vi "MultiScanDrift.vi"() -> ()   [LabVIEW 2021]
uses:
  shared/CorrelImages (SubVI)Single.vi
  <userlib>/Nanonis Prog Interface V5/Nanonis Prog Interface.lvlib
panel:
  in  "Lock-in":bool
  in  "Multipass":bool=TRUE
  in  "Add":bool=TRUE
  in  "end":sgl=-1.4 format="%#_6p"
  in  "step":sgl=0.2 format="%#_6p"
  in  "start":sgl=-2.0 format="%#_6p"
  in  "create Range":bool
  in  "PLL ON/OFF":bool
  in  "ref bias":dbl=-0.0012 format="%#_6p"
  in  "ref setpoint":bool
  in  "DC On":bool=TRUE
  out "Y drift":i32
  out "X drift":i32
  out "DC active\n(internal use)":bool
  in  "Drift correction Pixels":i32=180
  in  "Img Current":sgl=1e-10 format="%#_6p"
  in  "Img Bias (V) DC":sgl=1.0 format="%_2p"
  in  "Forward Speed":sgl=1.2e-09 format="%#_6p"
  in  "Backward Speed":sgl=8e-08 format="%#_6p"
  in  "Img Speed":sgl=4.5e-08 format="%#_6p"
  in  "Channel index (0-23)":u8(ring) items=["Current"=0, "Z (m)"=14]
  in  "Settling time (s)":dbl=0.7 format="%#_6p"
  in  "img bias":bool
  in  "img bias":dbl=-0.0012 format="%#_6p"
  in  "img delay (s)":u32=1
  out "tipLift":dbl format="%#_6p"
  in  "TipLiftList":i32(listbox)
  in  "Const Height":bool
  in  "CurrentList":i32(listbox)
  in  "BiasList":i32(listbox)
  out "Current":dbl=5e-11 format="%#_6p"
  out "Bias":dbl=0.02 format="%#_6p"
  # "Turn continuous scan off\n zero tiplift is '0'"
  # "Multipass Windows \nneeds to be open\n and OFF"
  # "5"
  # "10"
  # "15"
  # "20"
  # "25"
  # "30"
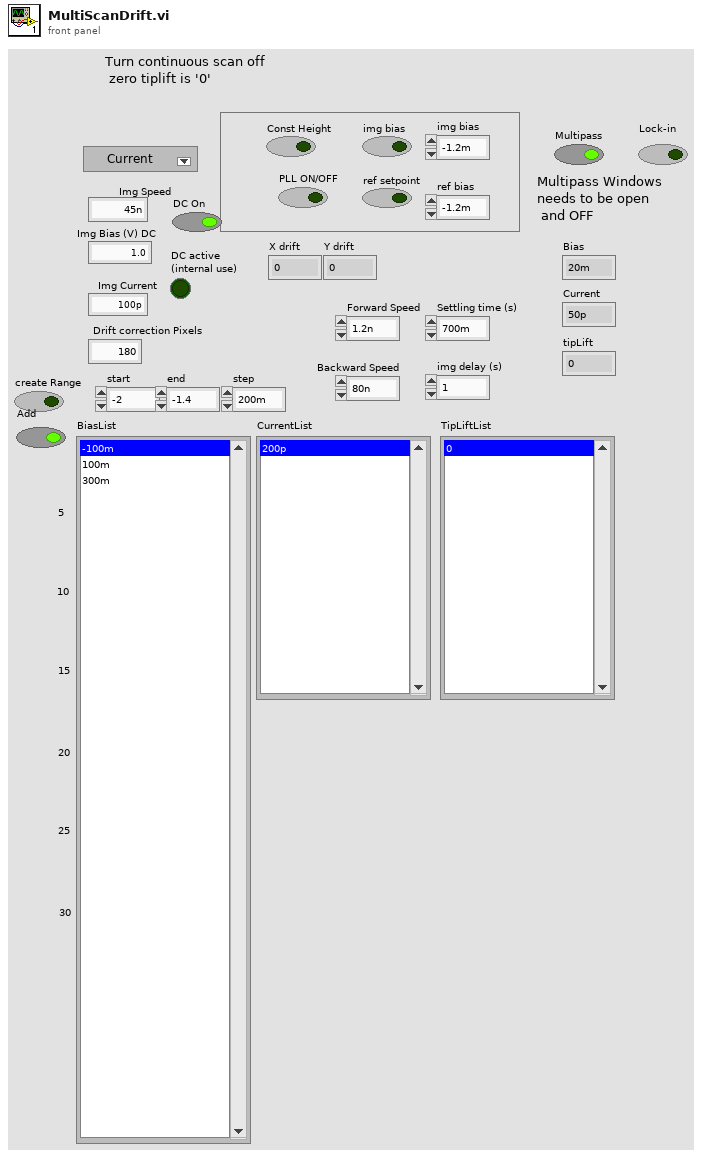
[diagram p1: front panel]
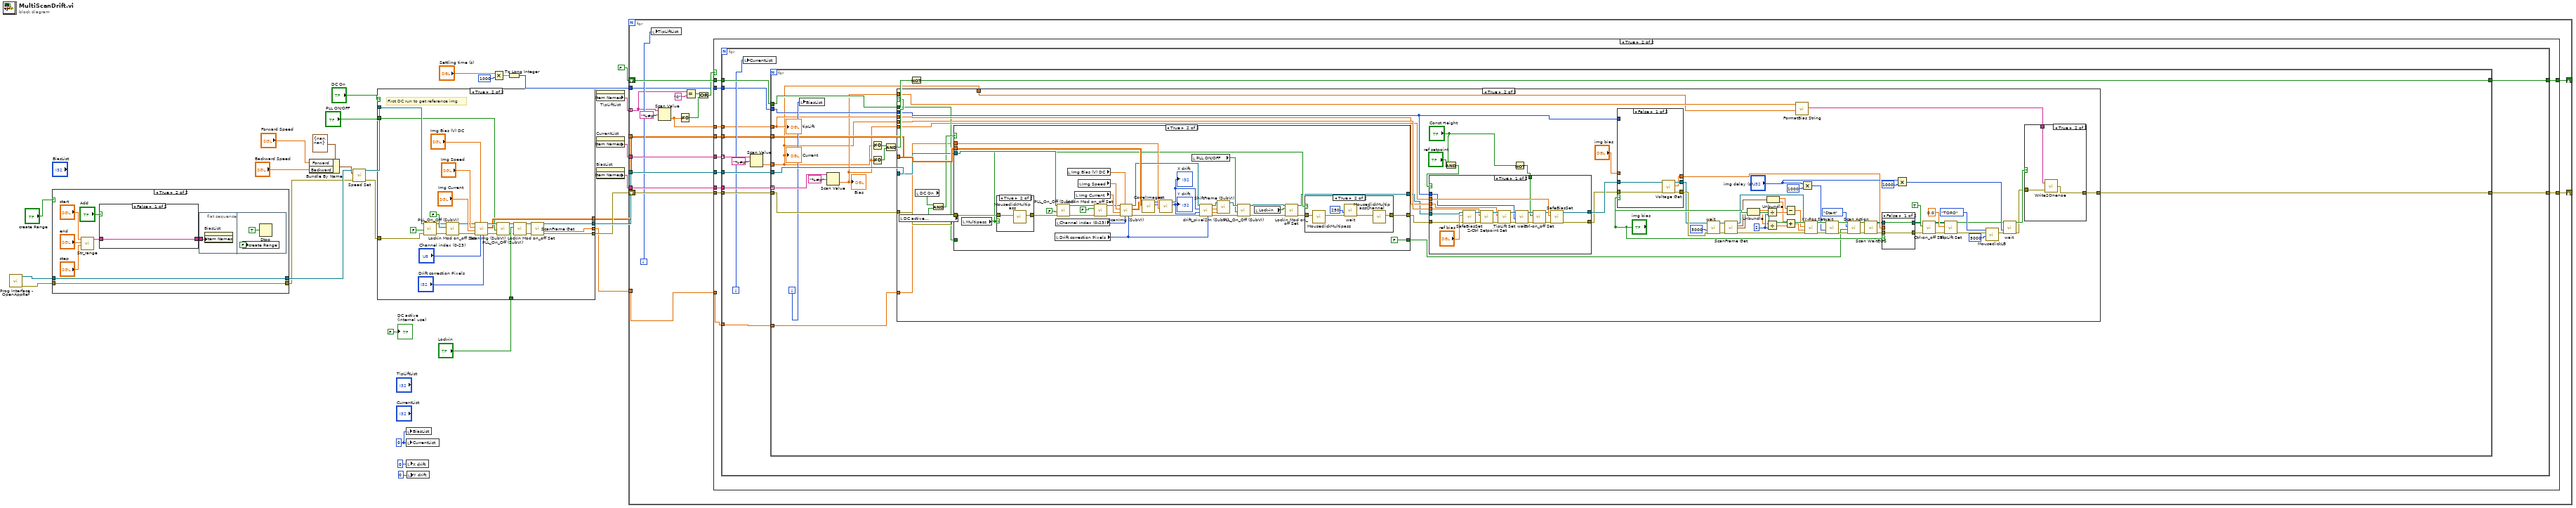
[diagram p0: block diagram]
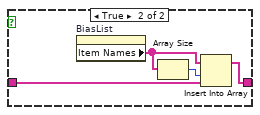
[diagram p3: hidden frame]
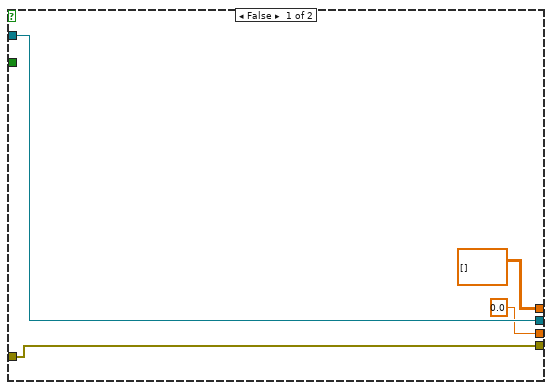
[diagram p4: hidden frame]
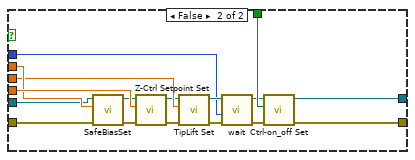
[diagram p7: hidden frame]
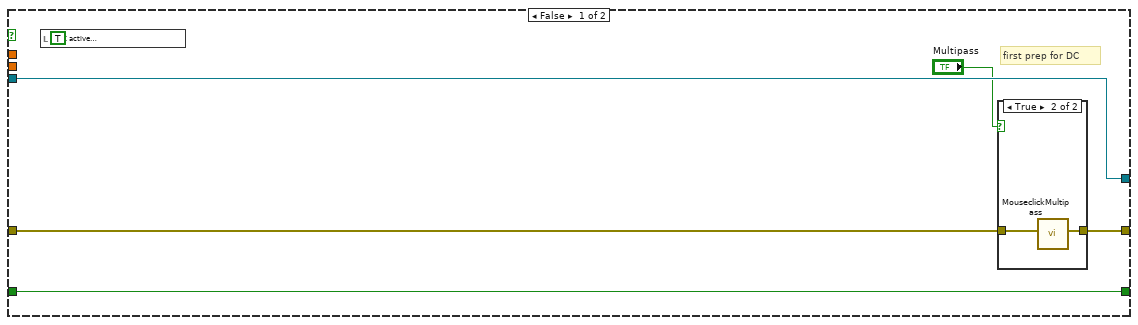
[diagram p9: hidden frame]
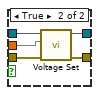
[diagram p13: hidden frame]
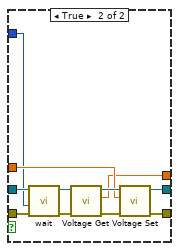
[diagram p14: hidden frame]
diagram:
  w30 = 0 ("BiasList")
  n1 = call <userlib>:"Prog Interface - OpenAppRef.vi"() -> ("Error out"=w3:errorcluster, "Application reference"=w5:refnum<vi>)  [unwired: 6 in]
  n2 = case shown="True" "create Range" {
    tunnel: w5 -> [w32 w40]
    tunnel: [w32 w40] -> w4
    tunnel: w3 -> [w31 w39]
    tunnel: [w31 w39] -> w2
    frame False {
    }
    frame True {
      n3 = call "Str_range.vi"("step"="step", "end"="end", "start"="start") -> ("Item Names"=w33:string[])  [unwired: 8 in]
      n4 = case shown="False" "Add" {
        tunnel: [w44 w46] -> w34
        tunnel: w33 -> [w44 w45]
        frame False {
        }
        frame True {
          n5 = property on="BiasList" class="LstBox (strict)"() -> ("Item Names"=w47:string[])  [unwired: 2 in, 2 out]
          n6 = Array Size(array=w47) -> (size(s)=w48:i32)
          n7 = Insert Into Array(array=w47, index=w48, new element=w45) -> (w46:string[])
        }
      }
      n8 = flat-sequence {
        tunnel: w34 -> [w41]
        frame #0 {
          n9 = property on="BiasList" class="LstBox (strict)"("Item Names"=w41) -> ()  [unwired: 2 in, 2 out]
        }
        frame #1 {
          n10 = local write "create Range"(FALSE ("Range")) -> ()
          n11 = Stop(stop? (T)=TRUE) -> ()
        }
      }
    }
  }
  n12 = Bundle By Name(cluster=cluster{"Forward":sgl, "Backward":sgl} {"Forward"=nan, "Backward"=nan} ("Speed (m/s)"), "Forward"="Forward Speed", "Backward"="Backward Speed") -> (w16:cluster{"Forward":sgl, "Backward":sgl})
  n13 = call <userlib>:"Speed Set.vi"("Application ref in"=w4, "Speed (m/s)"=w16, "error in (no error)"=w2) -> ("Application ref out"=w14:refnum<vi>, "error out"=w13:errorcluster)  [unwired: 11 in]
  n14 = case shown="True" "DC On" {
    tunnel: [w51 w66] -> w18
    tunnel: [w50 w65] -> w17
    tunnel: [dbl[][] [] ("Img") w71] -> w15
    tunnel: w14 -> [w51 w70]
    tunnel: w13 -> [w50 w69]
    tunnel: [sgl 0.0 ("Angle (deg)") w64] -> w8
    tunnel: "PLL ON/OFF" -> [_ w63]
    tunnel: "Lock-in" -> [_ w57]
    frame False {
    }
    frame True {
      # "First DC run to get reference img"
      n15 = call "PLL_On_Off (SubVI).vi"("error in (no error)"=w69, "Output ON/OFF (F=OFF)"=FALSE, "Application in"=w70) -> ("error out"=w59:errorcluster, "Application out"=w61:refnum<vi>)  [unwired: 7 in]
      n16 = call <userlib>:"Lockin Mod on_off Set.vi"("Error in (no error)"=w59, "Lockin ON/OFF"=FALSE, "Application ref in"=w61) -> ("Error out"=w58:errorcluster, "Application ref out"=w60:refnum<vi>)  [unwired: 7 in]
      n17 = call "ScanImg (SubVI).vi"("pixel"="Drift correction Pixels", "Channel index (0-23)"="Channel index (0-23)", "Bias (V)"="Img Bias (V) DC", "error in (no error)"=w58, "Current"="Img Current", "Img Speed"="Img Speed", "Application in"=w60) -> ("error out"=w74:errorcluster, "Img"=w71:dbl[][], "Application out"=w75:refnum<vi>)  [unwired: 2 in]
      n18 = call "PLL_On_Off (SubVI).vi"("error in (no error)"=w74, "Output ON/OFF (F=OFF)"=w63, "Application in"=w75) -> ("error out"=w56:errorcluster, "Application out"=w55:refnum<vi>)  [unwired: 7 in]
      n19 = call <userlib>:"Lockin Mod on_off Set.vi"("Error in (no error)"=w56, "Lockin ON/OFF"=w57, "Application ref in"=w55) -> ("Error out"=w53:errorcluster, "Application ref out"=w54:refnum<vi>)  [unwired: 7 in]
      n20 = call <userlib>:"ScanFrame Get.vi"("Application ref in"=w54, "error in (no error)"=w53) -> ("Application ref out"=w66:refnum<vi>, "Angle (deg)"=w64:sgl, "error out"=w65:errorcluster)  [unwired: 9 in, 2 out]
    }
  }
  n21 = local write "BiasList"(w30) -> ()
  n22 = local write "CurrentList"(w30) -> ()
  n23 = local write "X drift"(0 ("X drift")) -> ()
  n24 = local write "Y drift"(0 ("Y drift")) -> ()
  n25 = Multiply(x="Settling time (s)", y=u32 1000) -> (x*y=w26:dbl)
  n26 = To Long Integer(number=w26) -> (32bit integer=w27:i32)
  n27 = property on="TipLiftList" class="LstBox (strict)"() -> ("Item Names"=w22:string[])  [unwired: 2 in, 2 out]
  n28 = property on="CurrentList" class="LstBox (strict)"() -> ("Item Names"=w23:string[])  [unwired: 2 in, 2 out]
  n29 = property on="BiasList" class="LstBox (strict)"() -> ("Item Names"=w24:string[])  [unwired: 2 in, 2 out]
  n30 = for {
    tunnel: w24 -> [w94]
    tunnel: w23 -> [w93]
    tunnel: w18 -> [w92]
    tunnel: w22 -> [w88] mode=indexing
    shift-right: [w82] -> _
    shift-left: FALSE ("Direction: up/down (T=up)") -> [w95]
    tunnel: w27 -> [w81]
    tunnel: w15 -> [w80]
    tunnel: w8 -> [w79]
    shift-right: [w78] -> _
    shift-left: w17 -> [w91]
    i -> [w89]
    n31 = local write "TipLiftList"(w89) -> ()
    n32 = Scan Value(string=w88, format string="%#p") -> (value=w87:dbl)  [unwired: 1 in, 1 out]
    n33 = Not Equal To 0?(x=w87) -> (x != 0?=w86:bool)
    n34 = Equal?(x=w88, y="0") -> (x = y?=w83:bool)
    n35 = Or(x=w83, y=w86) -> (x .or. y?=w85:bool)
    n36 = case shown="True" w85 {
      tunnel: w95 -> [w97 w108]
      tunnel: w94 -> [_ w107]
      tunnel: w93 -> [_ w106]
      tunnel: w92 -> [_ w105]
      tunnel: w91 -> [w96 w104]
      tunnel: w87 -> [_ w103]
      tunnel: [w97 w102] -> w82
      tunnel: w81 -> [_ w101]
      tunnel: w80 -> [_ w100]
      tunnel: w79 -> [_ w99]
      tunnel: [w96 w98] -> w78
      frame False {
      }
      frame True {
        n37 = for {
          tunnel: w108 -> [w122]
          tunnel: w105 -> [w121]
          tunnel: w104 -> [w120]
          tunnel: w107 -> [w119]
          tunnel: w106 -> [w117] mode=indexing
          tunnel: w103 -> [w114]
          tunnel: [w113] -> w102
          tunnel: w101 -> [w112]
          tunnel: w100 -> [w111]
          tunnel: w99 -> [w110]
          tunnel: [w109] -> w98
          i -> [w115]
          n38 = local write "CurrentList"(w115) -> ()
          n39 = Scan Value(string=w117, format string="%#p") -> (value=w116:dbl)  [unwired: 1 in, 1 out]
          n40 = for {
            tunnel: w119 -> [w134] mode=indexing
            tunnel: w121 -> [w136]
            tunnel: w120 -> [w135]
            tunnel: w116 -> [w124]
            tunnel: w114 -> [w129]
            tunnel: w122 -> [w138]
            tunnel: [w137] -> w113
            tunnel: w112 -> [w128]
            tunnel: w111 -> [w127]
            tunnel: w110 -> [w126]
            tunnel: [w123] -> w109
            i -> [w130]
            n41 = local write "BiasList"(w130) -> ()
            n42 = Scan Value(string=w134, format string="%#p") -> (value=w125:dbl)  [unwired: 1 in, 1 out]
            "Bias" <- w125
            n43 = Not Equal To 0?(x=w124) -> (x != 0?=w133:bool)
            n44 = Not Equal To 0?(x=w125) -> (x != 0?=w132:bool)
            n45 = Compound Arithmetic op=AND(w133, w132) -> (w131:bool)
            n46 = case shown="True" w131 {
              tunnel: w138 -> [_ w180]
              tunnel: w125 -> [_ w210]
              tunnel: w136 -> [_ w187]
              tunnel: w135 -> [w140 w186]
              tunnel: w124 -> [_ w211]
              tunnel: w129 -> [_ w207]
              tunnel: w128 -> [_ w189]
              tunnel: w127 -> [_ w188]
              tunnel: w126 -> [_ w179]
              tunnel: w125 -> [_ w178]
              tunnel: w124 -> [_ w177]
              tunnel: [w140 w173] -> w123
              frame False {
              }
              frame True {
                w158 = 2
                n47 = local read "DC active\n(internal use)"() -> (w183:bool)
                n48 = local read "DC On"() -> (w182:bool)
                n49 = And(x=w182, y=w183) -> (x .and. y?=w181:bool)
                n50 = case shown="True" w181 {
                  tunnel: w188 -> [_ w298]
                  tunnel: w187 -> [w258 w288]
                  tunnel: w186 -> [w254 w277]
                  tunnel: [w253 w273] -> w185
                  tunnel: [w258 w263] -> w184
                  tunnel: [w256 FALSE ("Direction: up/down (T=up)")] -> w143
                  tunnel: w180 -> [w256 _]
                  tunnel: w179 -> [_ w283]
                  frame False {
                    # "first prep for DC"
                    n51 = local write "DC active\n(internal use)"(TRUE ("DC active")) -> ()
                    n52 = case shown="True" "Multipass" {
                      tunnel: w254 -> [w259 w261]
                      tunnel: [w259 w260] -> w253
                      frame False {
                      }
                      frame True {
                        n53 = call "MouseclickMultipass.vi"("error in (no error)"=w261) -> ("error out"=w260:errorcluster)  [unwired: 10 in]
                      }
                    }
                  }
                  frame True {
                    n54 = local read "Multipass"() -> (w272:bool)
                    n55 = case shown="True" w272 {
                      tunnel: w277 -> [w305 w307]
                      tunnel: [w305 w306] -> w276
                      frame False {
                      }
                      frame True {
                        n56 = call "MouseclickMultipass.vi"("error in (no error)"=w307) -> ("error out"=w306:errorcluster)  [unwired: 10 in]
                      }
                    }
                    n57 = local read "Drift correction Pixels"() -> (w285:i32)
                    n58 = local read "Channel index (0-23)"() -> (w293:u8)
                    n59 = call "PLL_On_Off (SubVI).vi"("error in (no error)"=w276, "Output ON/OFF (F=OFF)"=FALSE, "Application in"=w288) -> ("error out"=w270:errorcluster, "Application out"=w271:refnum<vi>)  [unwired: 7 in]
                    n60 = local read "Img Bias (V) DC"() -> (w294:sgl)
                    n61 = local read "Img Current"() -> (w295:sgl)
                    n62 = local read "Img Speed"() -> (w296:sgl)
                    n63 = call <userlib>:"Lockin Mod on_off Set.vi"("Error in (no error)"=w270, "Lockin ON/OFF"=FALSE, "Application ref in"=w271) -> ("Error out"=w268:errorcluster, "Application ref out"=w269:refnum<vi>)  [unwired: 7 in]
                    n64 = call "ScanImg (SubVI).vi"("pixel"=w285, "Channel index (0-23)"=w293, "Bias (V)"=w294, "error in (no error)"=w268, "Current"=w295, "Img Speed"=w296, "Application in"=w269) -> ("error out"=w275:errorcluster, "Img"=w297:dbl[][], "Application out"=w289:refnum<vi>)  [unwired: 2 in]
                    n65 = call-poly "CorrelImages.vi"("Ref Array"=w298, "New Image"=w297) -> ("Y drift"=w280:i32, "X drift"=w282:i32)  [unwired: 6 in, 2 out]
                    n66 = call "rot.vi"("angle"=w283, "y"=w280, "x"=w282) -> ("y'"=w279:i32, "x'"=w281:i32)  [unwired: 7 in]
                    "X drift" <- w281
                    "Y drift" <- w279
                    n67 = local read "PLL ON/OFF"() -> (w278:bool)
                    n68 = call "drift_pixel2m (SubVI).vi"("Application in"=w289, "X drift"=w281, "Y drift"=w279, "error in"=w275, "Drift correction Pixels"=w285) -> ("Application out"=w290:refnum<vi>, "x drift"=w292:sgl, "y drift"=w291:sgl, "error out"=w274:errorcluster)  [unwired: 1 in]
                    n69 = call "ShiftFrame (SubVI).vi"("Y shift"=w291, "X shift"=w292, "Application in"=w290) -> ("Application out"=w287:refnum<vi>)  [unwired: 8 in]
                    n70 = call "PLL_On_Off (SubVI).vi"("error in (no error)"=w274, "Output ON/OFF (F=OFF)"=w278, "Application in"=w287) -> ("error out"=w266:errorcluster, "Application out"=w264:refnum<vi>)  [unwired: 7 in]
                    n71 = local read "Lock-in"() -> (w262:bool)
                    n72 = call <userlib>:"Lockin Mod on_off Set.vi"("Error in (no error)"=w266, "Lockin ON/OFF"=w262, "Application ref in"=w264) -> ("Error out"=w265:errorcluster, "Application ref out"=w263:refnum<vi>)  [unwired: 7 in]
                    n73 = case shown="True" w272 {
                      tunnel: w265 -> [w299 w304]
                      tunnel: [w299 w303] -> w273
                      frame False {
                      }
                      frame True {
                        n74 = call "MouseclickMultipass.vi"("error in (no error)"=w304) -> ("error out"=w302:errorcluster)  [unwired: 10 in]
                        n75 = call "wait.vi"("error in"=w302, "milliseconds to wait"=u32 250) -> ("error out"=w301:errorcluster)  [unwired: 8 in, 1 out]
                        n76 = call "MouseclickMultipassChannel.vi"("error in (no error)"=w301) -> ("error out"=w303:errorcluster)  [unwired: 10 in]
                      }
                    }
                  }
                }
                n77 = And(x="Const Height", y="ref setpoint") -> (x .and. y?=w170:bool)
                n78 = Not(x="Const Height") -> (.not. x?=w209:bool)
                n79 = case shown="True" w170 {
                  tunnel: w211 -> [w218 w248]
                  tunnel: w210 -> [w231 w247]
                  tunnel: w209 -> [w225 w246]
                  tunnel: w207 -> [w219 w244]
                  tunnel: [w213 w243] -> w204
                  tunnel: [w212 w242] -> w203
                  tunnel: w189 -> [w220 w238]
                  tunnel: w185 -> [w216 w237]
                  tunnel: w184 -> [w217 w236]
                  frame True {
                    n80 = call "SafeBiasSet.vi"("Application ref in"=w217, "Bias (V)"="ref bias", "error in (no error)"=w216) -> ("Application ref out"=w228:refnum<vi>, "Error out"=w230:errorcluster)  [unwired: 6 in]
                    n81 = call <userlib>:"Z-Ctrl Setpoint Set.vi"("error in (no error)"=w230, "Z Controller setpoint"=w218, "Application ref in"=w228) -> ("error out"=w222:errorcluster, "Application ref out"=w224:refnum<vi>)  [unwired: 7 in]
                    n82 = call <userlib>:"TipLift Set.vi"("error in (no error)"=w222, "TipLift (m)"=w219, "Application ref in"=w224) -> ("error out"=w221:errorcluster, "Application ref out"=w223:refnum<vi>)  [unwired: 7 in]
                    n83 = call "wait.vi"("error in"=w221, "milliseconds to wait"=w220, "application reference in"=w223) -> ("error out"=w227:errorcluster, "application reference out"=w226:refnum<vi>)  [unwired: 7 in]
                    n84 = call <userlib>:"Ctrl-on_off Set.vi"("error in (no error)"=w227, "Z Controller ON/OFF"=w225, "Application ref in"=w226) -> ("error out"=w214:errorcluster, "Application ref out"=w215:refnum<vi>)  [unwired: 7 in]
                    n85 = call "SafeBiasSet.vi"("Application ref in"=w215, "Bias (V)"=w231, "error in (no error)"=w214) -> ("Application ref out"=w213:refnum<vi>, "Error out"=w212:errorcluster)  [unwired: 6 in]
                  }
                  frame False {
                    n86 = call "SafeBiasSet.vi"("Application ref in"=w236, "Bias (V)"=w247, "error in (no error)"=w237) -> ("Application ref out"=w235:refnum<vi>, "Error out"=w234:errorcluster)  [unwired: 6 in]
                    n87 = call <userlib>:"Z-Ctrl Setpoint Set.vi"("error in (no error)"=w234, "Z Controller setpoint"=w248, "Application ref in"=w235) -> ("error out"=w232:errorcluster, "Application ref out"=w233:refnum<vi>)  [unwired: 7 in]
                    n88 = call <userlib>:"TipLift Set.vi"("error in (no error)"=w232, "TipLift (m)"=w244, "Application ref in"=w233) -> ("error out"=w239:errorcluster, "Application ref out"=w245:refnum<vi>)  [unwired: 7 in]
                    n89 = call "wait.vi"("error in"=w239, "milliseconds to wait"=w238, "application reference in"=w245) -> ("error out"=w240:errorcluster, "application reference out"=w241:refnum<vi>)  [unwired: 7 in]
                    n90 = call <userlib>:"Ctrl-on_off Set.vi"("error in (no error)"=w240, "Z Controller ON/OFF"=w246, "Application ref in"=w241) -> ("error out"=w242:errorcluster, "Application ref out"=w243:refnum<vi>)  [unwired: 7 in]
                  }
                }
                n91 = case shown="False" "img bias" {
                  tunnel: w204 -> [w319 w321]
                  tunnel: [w318 w328] -> w141
                  tunnel: w203 -> [w315 w324]
                  tunnel: [w316 w327] -> w142
                  tunnel: "img bias" -> [_ w326]
                  tunnel: [w317 w325] -> w201
                  tunnel: w189 -> [_ w320]
                  frame False {
                    n92 = call <userlib>:"Voltage Get.vi"("error in (no error)"=w315, "Application ref in"=w319) -> ("error out"=w316:errorcluster, "Bias (V)"=w317:sgl, "Application ref out"=w318:refnum<vi>)  [unwired: 7 in]
                  }
                  frame True {
                    n93 = call "wait.vi"("error in"=w324, "milliseconds to wait"=w320, "application reference in"=w321) -> ("error out"=w323:errorcluster, "application reference out"=w322:refnum<vi>)  [unwired: 7 in]
                    n94 = call <userlib>:"Voltage Get.vi"("error in (no error)"=w323, "Application ref in"=w322) -> ("error out"=w330:errorcluster, "Bias (V)"=w325:sgl, "Application ref out"=w329:refnum<vi>)  [unwired: 7 in]
                    n95 = call <userlib>:"Voltage Set.vi"("Error in (no error)"=w330, "Bias (V)"=w326, "Application ref in"=w329) -> ("Error out"=w327:errorcluster, "Application ref out"=w328:refnum<vi>)  [unwired: 7 in]
                  }
                }
                n96 = call "wait.vi"("error in"=w142, "milliseconds to wait"=u32 3000 ("y"), "application reference in"=w141) -> ("error out"=w150:errorcluster, "application reference out"=w149:refnum<vi>)  [unwired: 7 in]
                n97 = call <userlib>:"ScanFrame Get.vi"("Application ref in"=w149, "error in (no error)"=w150) -> ("Application ref out"=w169:refnum<vi>, "Center coordinates (m)"=w153:cluster{"Xc":sgl, "Yc":sgl}, "Size (m)"=w154:cluster{"Width":sgl, "Height":sgl}, "error out"=w168:errorcluster)  [unwired: 9 in, 1 out]
                n98 = Unbundle(w154) -> ("Width"=w156:sgl, "Height"=w157:sgl)
                n99 = Divide(x=w156, y=w158) -> (x/y=w160:sgl)
                n100 = Divide(x=w157, y=w158) -> (x/y=w159:sgl)
                n101 = Unbundle(w153) -> ("Xc"=w161:sgl, "Yc"=w155:sgl)
                n102 = Subtract(x=w161, y=w160) -> (x-y=w162:sgl)
                n103 = Add(x=w155, y=w159) -> (x+y=w163:sgl)
                n104 = call "FormatBias String.vi"("current"=w177, "bias"=w178) -> ("resulting string"=w174:string)  [unwired: 9 in]
                n105 = Multiply(x="img delay (s)", y=u32 1000) -> (x*y=w165:u32)
                n106 = call <userlib>:"XY-Pos Set.vi"("error in (no error)"=w168, "Y (m)"=w163, "X (m)"=w162, "Application ref in"=w169) -> ("error out"=w167:errorcluster, "Application ref out"=w166:refnum<vi>)  [unwired: 4 in]
                n107 = call "wait.vi"("error in"=w167, "milliseconds to wait"=w165, "application reference in"=w166) -> ("error out"=w147:errorcluster, "application reference out"=w148:refnum<vi>)  [unwired: 7 in]
                n108 = call <userlib>:"Scan Action.vi"("error in (no error)"=w147, "Direction: up/down (T=up)"=w143, "Scan action (Start)"=enum16{"Start", "Stop", "Pause", "Resume"}."Start", "Application ref in"=w148) -> ("error out"=w145:errorcluster, "Application ref out"=w146:refnum<vi>)  [unwired: 5 in]
                n109 = call <userlib>:"Scan WaitEOS.vi"("error in (no error)"=w145, "Application ref in"=w146) -> ("error out"=w199:errorcluster, "Application ref out"=w200:refnum<vi>)  [unwired: 5 in, 2 out]
                n110 = case shown="False" "img bias" {
                  tunnel: w200 -> [w309 w312]
                  tunnel: [w309 w314] -> w198
                  tunnel: [w308 w313] -> w197
                  tunnel: w199 -> [w308 w311]
                  tunnel: w201 -> [_ w310]
                  frame False {
                  }
                  frame True {
                    n111 = call <userlib>:"Voltage Set.vi"("Error in (no error)"=w311, "Bias (V)"=w310, "Application ref in"=w312) -> ("Error out"=w313:errorcluster, "Application ref out"=w314:refnum<vi>)  [unwired: 7 in]
                  }
                }
                n112 = Multiply(x="img delay (s)", y=u32 1000) -> (x*y=w191:u32)
                n113 = call <userlib>:"Ctrl-on_off Set.vi"("error in (no error)"=w197, "Z Controller ON/OFF"=TRUE, "Application ref in"=w198) -> ("error out"=w196:errorcluster, "Application ref out"=w195:refnum<vi>)  [unwired: 7 in]
                n114 = call <userlib>:"TipLift Set.vi"("error in (no error)"=w196, "TipLift (m)"=sgl 0.0, "Application ref in"=w195) -> ("error out"=w206:errorcluster)  [unwired: 7 in, 1 out]
                n115 = call "MouseclickLB.vi"("nMilliseconds"=5000, "error in (no error)"=w206, "Click"=enum16{"Header", "TOPO", "STS", "GRID"}."TOPO") -> ("error out"=w190:errorcluster)  [unwired: 8 in]
                n116 = call "wait.vi"("error in"=w190, "milliseconds to wait"=w191) -> ("error out"=w175:errorcluster)  [unwired: 8 in, 1 out]
                n117 = case shown="True" "img bias" {
                  tunnel: w175 -> [w249 w252]
                  tunnel: w174 -> [_ w251]
                  tunnel: [w249 w250] -> w173
                  frame False {
                  }
                  frame True {
                    n118 = call "Write2Onenoe.vi"("error in (no error)"=w252, "strSendText"=w251) -> ("error out"=w250:errorcluster)
                  }
                }
              }
            }
            n119 = Not(x=w138) -> (.not. x?=w137:bool)
            "Current" <- w124
            "tipLift" <- w129
          }
        }
      }
    }
  }
  "DC active\n(internal use)" <- FALSE ("DC active")
